vi "Teleop.vi"(10 "Match Info":T5={"Autonomous Elapsed Seconds"=0.0, "TeleOp Elapsed Seconds"=0.0, "Disabled Elapsed Seconds"=0.0, "Visited Autonomous"=FALSE, "Visited TeleOp"=FALSE, "Visited Disabled"=FALSE, "Autonomous Settings"={"Autonomous Style"=enum."Independent", "VI Refnum"=refnum}}, 11 "Call Context":T6) -> ()   [LabVIEW 2020]
doc: "This VI is called for each TeleOp packet received from the DS where the robot is not disabled. It is often used to read from the joysticks and update I/O or to update setpoints for timed control loops. It should complete and return within 20 milliseconds or it may miss DS packets."
uses:
  <vilib>/Rock Robotics/WPI/DriverStation/WPI_DriverStationDerivedRobotMode.ctl
  <vilib>/Rock Robotics/WPI/DriverStation/WPI_DriverStationMatch Info.ctl
  <vilib>/Rock Robotics/WPI/Solenoid/WPI_SolenoidValue.ctl
  <vilib>/Rock Robotics/WPI/ThirdParty/Phoenix-LabVIEW/CANCoder/Controls/CTRE_Phoenix_CANcoder_Faults.ctl
  <vilib>/Rock Robotics/WPI/ThirdParty/Phoenix-LabVIEW/CANCoder/Controls/CTRE_Phoenix_CANcoder_StatusFrame.ctl
  <vilib>/Rock Robotics/WPI/ThirdParty/Phoenix-LabVIEW/Motor Controller/Controls/CTRE_Phoenix_MotorControl_ControlMode.ctl
  <vilib>/Rock Robotics/Network Tables/NT Read Boolean.vi
  <vilib>/Rock Robotics/Network Tables/NT Read Number.vi
  <vilib>/Rock Robotics/WPI/Utilities/WPI_GetSetVariantRefNum.vi
  <vilib>/Rock Robotics/Network Tables/NT Write Boolean Array.vi
  <vilib>/Rock Robotics/Network Tables/NT Write Numeric Array.vi
  <vilib>/Rock Robotics/WPI/Solenoid/WPI_SolenoidSetEnum.vi
  <vilib>/Rock Robotics/WPI/ThirdParty/Phoenix-LabVIEW/CANCoder/Get/CTRE_Phoenix_CANcoder_GetSensorData.vi
  <vilib>/Rock Robotics/WPI/ThirdParty/Phoenix-LabVIEW/Motor Controller/Get/CTRE_Phoenix_MotorController_GetSelectedSensorData.vi
  <vilib>/Rock Robotics/WPI/RobotDrive/WPI_RobotDriveArcadeDrive_Standard(NoSaturation).vi
  <vilib>/Rock Robotics/WPI/ThirdParty/Phoenix-LabVIEW/CANCoder/Set/CTRE_Phoenix_CANcoder_SetPosition.vi
panel:
  out "Talon FX Left Encoder":i32
  out "Talon FX Right Encoder":i32
  out "Right Encoder Position":dbl=-0.5 format="%#_13g"
  out "Left Encoder Position":dbl format="%#_13g"
  out "periodMs":u32=1
  in  "Get status":bool=TRUE
  in  "CANcoder Status Frame":T1=267264 items=["SensorData"=267264, "VbatAndFaults"=267328]
  in  "Period (ms)":u8
  out "In Starting Lvl Seq":bool
  out "In High Lvl Seq":bool
  out "In Ground Lvl Seq":bool
  out "In Mid Lvl Seq":bool
  out "Set Arm Angle Rate":dbl format="%#_13g"
  out "Arm Elevation Position":dbl
  out "Arm Telescope Position":dbl format="%#_13g"
  out "Set Arm Tellescope Rate":dbl
  in  "Arm Tellescope Ground Set Point":dbl=780.0
  in  "Arm Tellescope Allowed Error":dbl=30.0 format="%#_13g"
  in  "Arm Elevation Ground Set Point":dbl=46.0 format="%#_13g"
  in  "Arm Elevation Allowed Error":dbl=3.0 format="%#_13g"
  in  "Arm Tellescope Mid Set Point":dbl=1130.0
  in  "Arm Elevation Mid Setpoint":dbl=80.0 format="%#_13g"
  in  "Arm Tellescope High Set Point":dbl=1790.0
  in  "Arm Elevation High Set Point":dbl=95.0 format="%#_13g"
  in  "Arm Elevation Starting position Set Point":dbl=5.0
  in  "Arm Telescope Starting Set Point":dbl=30.0
  out "Arrived in Set Location":bool
  out "Sticky Faults":T2={"Hardware Fault"=FALSE, "API Error"=FALSE, "Under Voltage"=FALSE, "Reset During Enable"=FALSE, "Magnet Too Weak"=TRUE}
  out "Faults":T3
  in  "Intake value":dbl format="%#_13g"
  in  "Turn Shifter Off":T4=enum."Reverse"
  in  "Shifter Turn On":T4=enum."Forward"
  in  "Break Turn Off":T4=enum."Reverse"
  in  "Break Turn On":T4=enum."Forward"
  out "Sample Slider 0":dbl(slide) scale=0.0..5.0
  out "Sample Boolean 1":bool
  out "Sample Boolean 0":bool
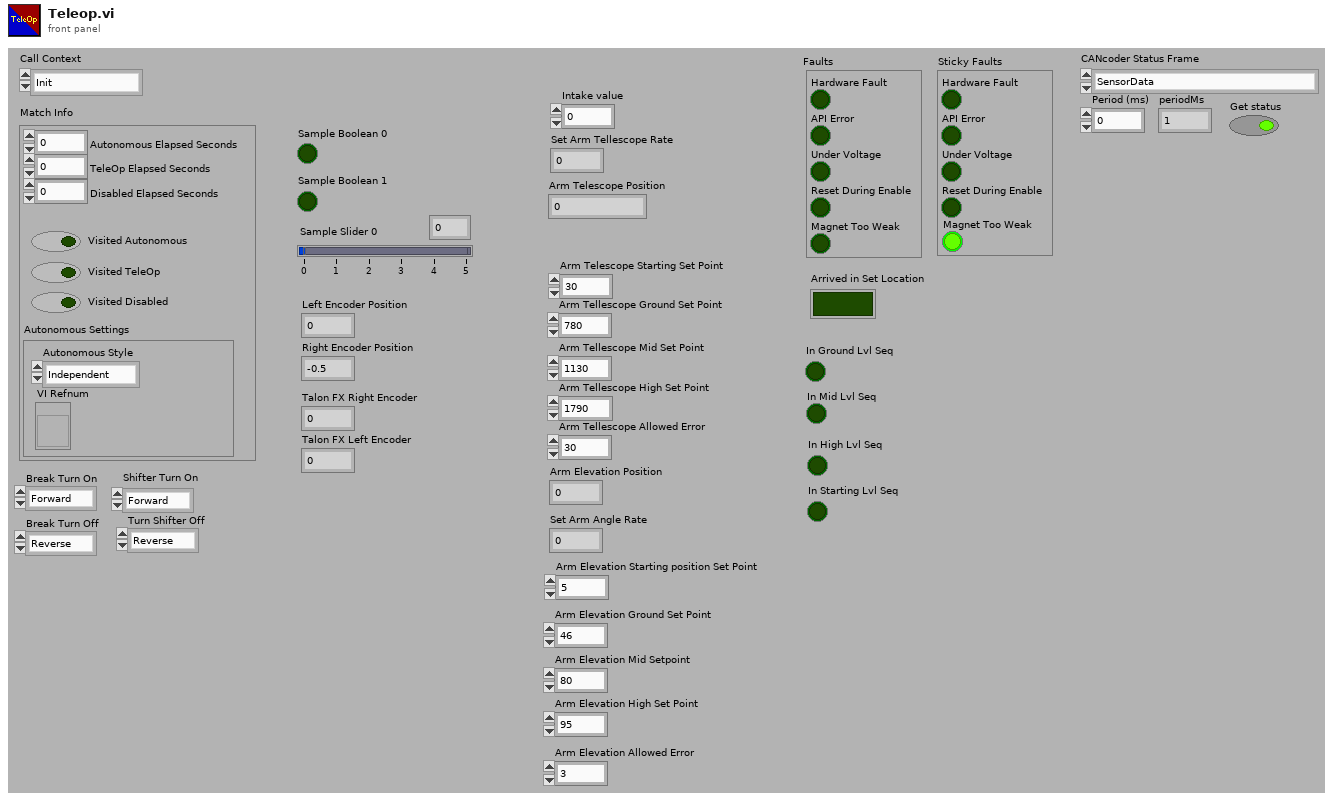
[diagram p1: front panel]
types:
  T1 = typedef "CTRE_Phoenix_CANcoder_StatusFrame.ctl" = u32
  T2 = cluster{"Hardware Fault":bool, "API Error":bool, "Under Voltage":bool, "Reset During Enable":bool, "Magnet Too Weak":bool}
  T3 = typedef "CTRE_Phoenix_CANcoder_Faults.ctl" = cluster{"Hardware Fault":bool, "API Error":bool, "Under Voltage":bool, "Reset During Enable":bool, "Magnet Too Weak":bool}
  T4 = typedef "WPI_SolenoidValue.ctl" = enum16{"Off", "On", "Forward", "Reverse"}
  T5 = typedef "WPI_DriverStationMatch Info.ctl" = cluster{"Autonomous Elapsed Seconds":dbl, "TeleOp Elapsed Seconds":dbl, "Disabled Elapsed Seconds":dbl, "Visited Autonomous":bool, "Visited TeleOp":bool, "Visited Disabled":bool, "Autonomous Settings":cluster{"Autonomous Style":enum16{"Iterative", "Independent"}, "VI Refnum":refnum<vi>}}
  T6 = typedef "WPI_DriverStationDerivedRobotMode.ctl" = enum16{"Init", "Execute", "Stop"}
  T7 = typedef "CTRE_Phoenix_MotorControl_ControlMode.ctl" = u16
  T8 = typedef "CTRE_Phoenix_CANcoder_DeviceRef.ctl" = cluster{"DeviceStatus":errorcluster, "Device Number":u8, "Handle":u64, "UsageFrame":u32, "Library Path":path}
  T9 = typedef "WPI_EncoderDevRef.ctl" = cluster{"DevStatus":errorcluster, "EncoderIndex":T10, "CounterIndex":T11, "DistancePerCount":dbl, "Decoding Type":T12}
  T10 = typedef "FPGA_EncoderIdx.ctl" = enum8{"Enc 0", "Enc 1", "Enc 2", "Enc 3", "Enc 4", "Enc 5", "Enc 6", "Enc 7", "Invalid"}
  T11 = typedef "FPGA_CounterCtrSystemIndex.ctl" = enum8{"Ctr 0", "Ctr 1", "Ctr 2", "Ctr 3", "Ctr 4", "Ctr 5", "Ctr 6", "Ctr 7", "Invalid"}
  T12 = typedef "WPI_EncoderType.ctl" = enum16{"1x", "2x", "4x"}
  T13 = typedef "WPI_MotorControlDeviceRef.ctl" = cluster{"DeviceStatus":errorcluster, "Type":T14, "PWM":cluster{"PWM Channel":T15, "DeadBand":T16}, "CAN":cluster{"Device Number":u8, "SetOutput VI Ref":variant, "GetOutput VI Ref":variant, "Enable VI Ref":variant, "Disable VI Ref":variant, "Data":variant}, "Invert":bool, "DIO PWM":cluster{"PWM \"Enable\" Channel":T15, "DIOChannel":T17, "PWM Rate":dbl}}
  T14 = typedef "WPI_MotorControlType.ctl" = enum16{"PWM", "CAN", "DIO PWM"}
  T15 = typedef "FPGA_DIOPWMChannel.ctl" = enum8{"PWM 0", "PWM 1", "PWM 2", "PWM 3", "PWM 4", "PWM 5", "PWM 6", "PWM 7", "PWM 8", "PWM 9", "PWM MXP 0", "PWM MXP 1", "PWM MXP 2", "PWM MXP 3", "PWM MXP 4", "PWM MXP 5", "PWM MXP 6", "PWM MXP 7", "PWM MXP 8", "PWM MXP 9", "Invalid"}
  T16 = typedef "WPI_PWMDeadband.ctl" = cluster{"Name":string, "maxPositivePwm":i32, "minPositivePwm":i32, "centerPwm":i32, "maxNegativePwm":i32, "minNegativePwm":i32, "angularRange":u16}
  T17 = typedef "FPGA_DIOChannel.ctl" = enum8{"DIO 0", "DIO 1", "DIO 2", "DIO 3", "DIO 4", "DIO 5", "DIO 6", "DIO 7", "DIO 8", "DIO 9", "DIO MXP 0", "DIO MXP 1", "DIO MXP 2", "DIO MXP 3", "DIO MXP 4", "DIO MXP 5", "DIO MXP 6", "DIO MXP 7", "DIO MXP 8", "DIO MXP 9", "DIO MXP 10", "DIO MXP 11", "DIO MXP 12", "DIO MXP 13", "DIO MXP 14", "DIO MXP 15", "SPI Port CS1", "SPI Port CS2", "SPI Port CS3", "SPI Port MISO", "SPI Port MOSI", "Invalid"}
  T18 = typedef "WPI_JoystickDevRef.ctl" = cluster{"Device":T19}
  T19 = typedef "WPI_JoystickDeviceEnum.ctl" = enum16{"USB 0", "USB 1", "USB 2", "USB 3", "USB 4", "USB 5"}
  T20 = typedef "WPI_RobotDriveDevRef.ctl" = cluster{"DevStatus":errorcluster, "Motors[]":T13[], "Square Inputs":bool, "Max Output":dbl}
  T21 = typedef "WPI_ServoDeviceRef.ctl" = cluster{"DeviceStatus":errorcluster, "PWM Channel":T15, "DeadBand":T16}
  T22 = typedef "WPI_SolenoidDevRef.ctl" = cluster{"DevStatus":errorcluster, "Pneumatics Control Module":u8, "Forward Solenoid Channel":T23, "Reverse Solenoid Channel":T23}
  T23 = typedef "WPI_SolenoidChannel.ctl" = enum8{"Solenoid 0", "Solenoid 1", "Solenoid 2", "Solenoid 3", "Solenoid 4", "Solenoid 5", "Solenoid 6", "Solenoid 7", "Solenoid 8", "Solenoid 9", "Solenoid 10", "Solenoid 11", "Solenoid 12", "Solenoid 13", "Solenoid 14", "Solenoid 15", "Invalid"}
  T24 = typedef "WPI_SwitchDevRef.ctl" = cluster{"DevStatus":errorcluster, "DIO Channel":T17, "CntIndex":T11, "Normally Closed":bool}
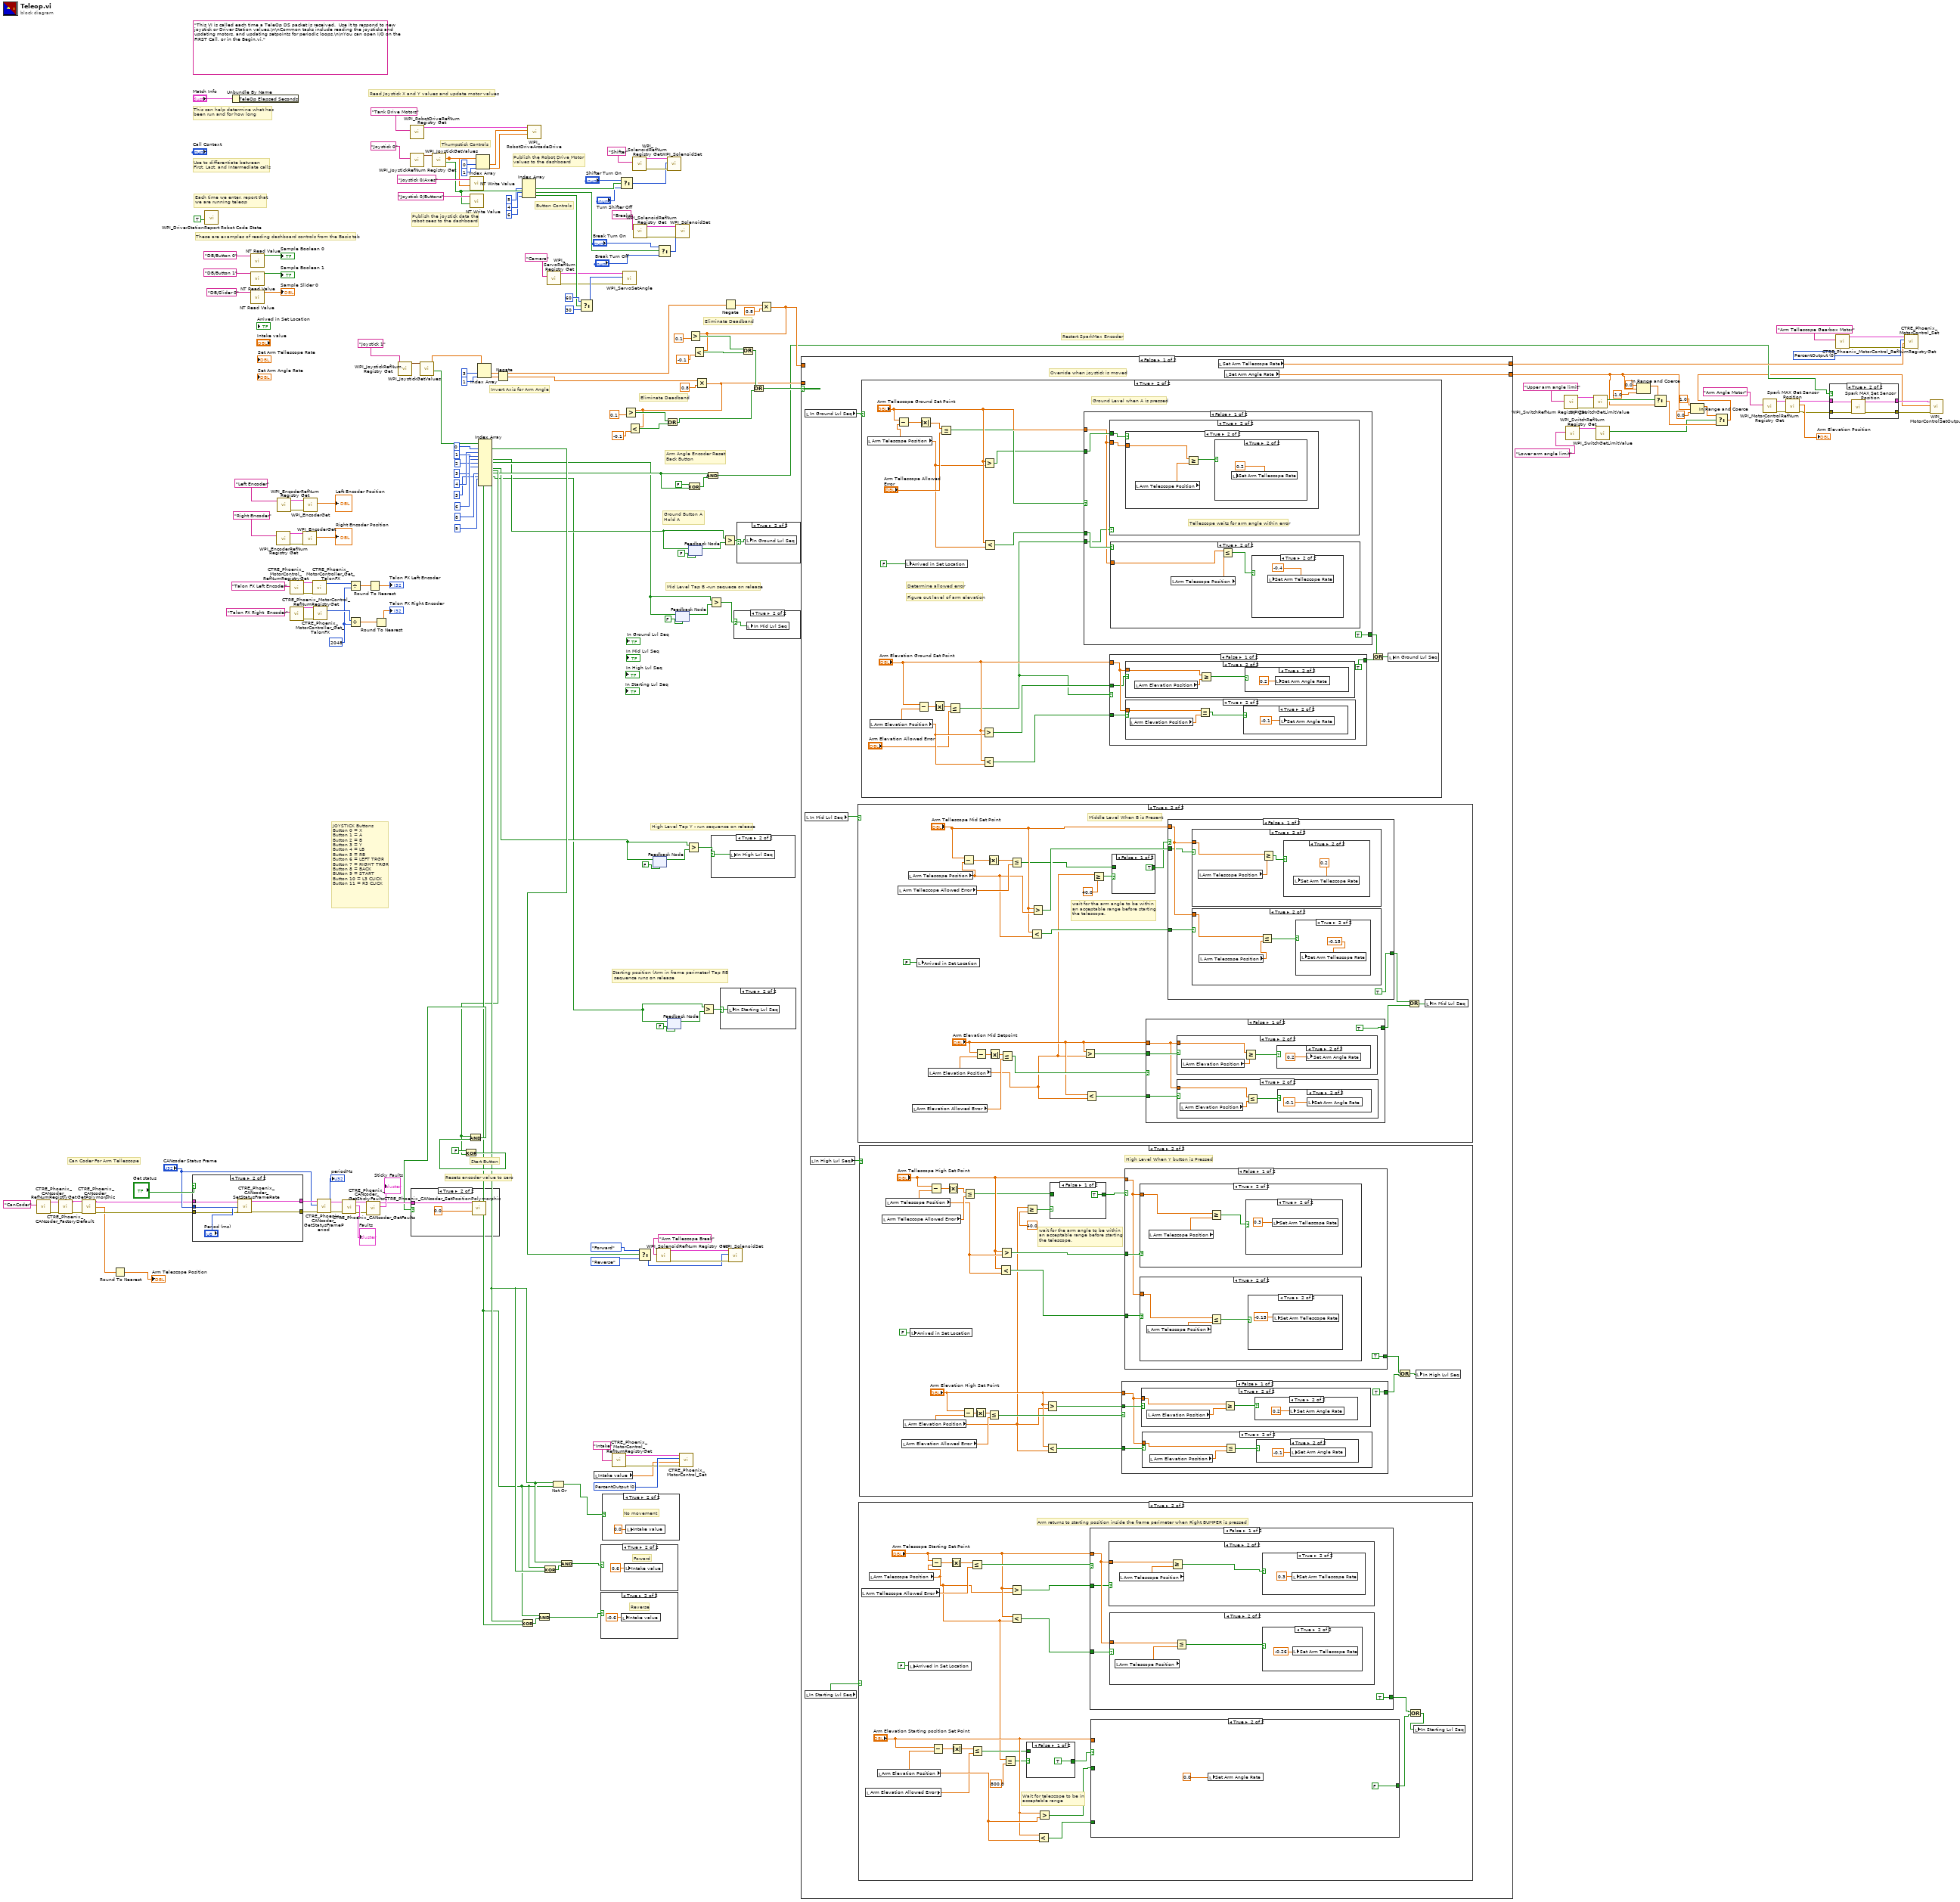
[diagram p0: block diagram]
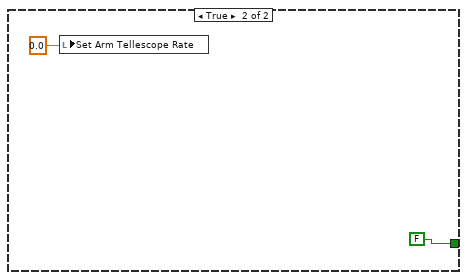
[diagram p15: hidden frame]
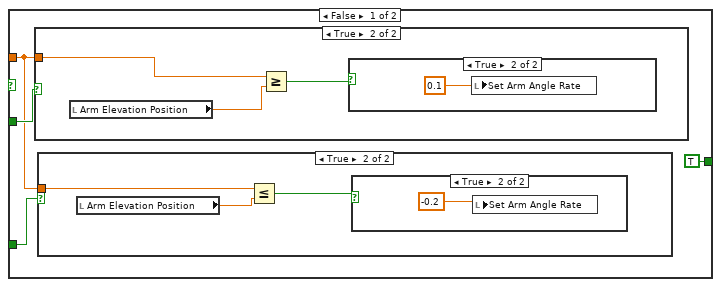
[diagram p16: hidden frame]
diagram:
  w11 = 2048 ("y")
  w144 = T7 0 items=["PercentOutput"=0, "Position"=1, "Velocity"=2, "Current"=3, "Follower"=5, "MotionProfile"=6, "MotionMagic"=7, "MotionProfileArc"=10, "Disabled"=15] ("Control Mode")
  w149 = T7 0 items=["PercentOutput"=0, "Position"=1, "Velocity"=2, "Current"=3, "Follower"=5, "MotionProfile"=6, "MotionMagic"=7, "MotionProfileArc"=10, "Disabled"=15] ("Control Mode")
  (unwired) "This VI is called each time a TeleOp DS packet is received.  Use it to respond to new joystick or Driver Station values.\n\nCommon tasks include reading the joysticks and updating motors, and updating setpoints for periodic loops.\n\nYou can open I/O on the FIRST Call, or in the Begin.vi."
  # "Can Coder For Arm Tellescope"
  # "Starting position (Arm in frame perimeter) Tap RB\n sequence runs on release"
  # "Mid Level Tap B -run sequece on release"
  # "Arm Angle Encoder Reset\nBack Button"
  # "Restart SparkMax Encoder"
  # "Invert Axis for Arm Angle"
  # "Eliminate Deadband"
  # "High Level Tap Y - run sequence on release"
  # "Ground Button A\nHold A"
  # "Start Button"
  # "Resets encoder value to zero"
  # "Eliminate Deadband"
  # "JOYSTICK Buttons\nButton 0 = X\nButton 1 = A\nButton 2 = B\nButton 3 = Y\nButton 4 = LB \nButton 5 = RB\nButton 6 = LEFT TRGR \nButton 7 = RIGHT TRGR \nButton 8 = BACK\nBUtton 9 = START\nButton 10 = L3 CLICK\nButton 11 = R3 CLICK"
  # "Thumpstick Controls"
  # "Button Controls"
  # "Publish the Robot Drive Motor\nvalues to the dashboard"
  # "Publish the joystick data the\nrobot sees to the dashboard"
  # "Read Joystick X and Y values and update motor values"
  # "These are examples of reading dashboard controls from the Basic tab"
  # "Each time we enter, report that\nwe are running teleop"
  # "Use to differentiate between\nFirst, Last, and Intermediate calls"
  # "This can help determine what has\nbeen run and for how long"
  n1 = call <vilib>:"CTRE_Phoenix_CANcoder_RefNumRegistryGet.vi"("refnum name"="CanCoder") -> ("error out"=w41:errorcluster, "CTRE_CANcoder_DeviceRef"=w40:T8)  [unwired: 9 in]
  n2 = call <vilib>:"CTRE_Phoenix_CANcoder_FactoryDefault.vi"("error in"=w41, "CTRE_CANcoder_DeviceRef"=w40) -> ("error out"=w39:errorcluster, "CTRE_CANcoder_DeviceRef"=w38:T8)  [unwired: 8 in]
  n3 = call-poly <vilib>:"CTRE_Phoenix_CANcoder_GetPolymorphic.vi"("CTRE_CANcoder_DeviceRef"=w38, "error in"=w39) -> ("CTRE_CANcoder_DeviceRef"=w36:T8, "Position"=w35:dbl, "error out"=w37:errorcluster)  [unwired: 9 in, 2 out]
  n4 = Round To Nearest(number=w35) -> (nearest integer value=→"Arm Telescope Position":dbl)
  n5 = case shown="True" "Get status" {
    tunnel: w36 -> [w194 w200]
    tunnel: "CANcoder Status Frame" -> [_ w199]
    tunnel: [w194 w197] -> w45
    tunnel: [w193 w196] -> w44
    tunnel: w37 -> [w193 w195]
    frame False {
    }
    frame True {
      n6 = call <vilib>:"CTRE_Phoenix_CANcoder_SetStatusFrameRate.vi"("error in (no error)"=w195, "Period (ms)"="Period (ms)", "CANcoder Status Frame"=w199, "CTRE_CANcoder_DeviceRef"=w200) -> ("error out"=w196:errorcluster, "CTRE_CANcoder_DeviceRef"=w197:T8)  [unwired: 6 in]
    }
  }
  n7 = call <vilib>:"WPI_DriverStationReport Robot Code State.vi"("TeleOp"=TRUE ("Autonomous")) -> ()  [unwired: 10 in, 1 out]
  n8 = Unbundle By Name("Match Info") -> ()  [unwired: 1 out]
  n9 = call-poly <vilib>:"NT Read Value.vi"("name"="DB/Button 0" ("refnum name")) -> ("value"=→"Sample Boolean 0":bool)  [unwired: 8 in, 2 out]
  n10 = call-poly <vilib>:"NT Read Value.vi"("name"="DB/Slider 0" ("refnum name")) -> ("value"=→"Sample Slider 0":dbl)  [unwired: 8 in, 2 out]
  n11 = call-poly <vilib>:"NT Read Value.vi"("name"="DB/Button 1" ("refnum name")) -> ("value"=→"Sample Boolean 1":bool)  [unwired: 8 in, 2 out]
  n12 = call <vilib>:"WPI_EncoderRefNum Registry Get.vi"("refnum name"="Right Encoder") -> ("error out"=w27:errorcluster, "EncoderDevRef"=w26:T9)  [unwired: 9 in]
  n13 = call <vilib>:"WPI_EncoderRefNum Registry Get.vi"("refnum name"="Left Encoder") -> ("error out"=w30:errorcluster, "EncoderDevRef"=w29:T9)  [unwired: 9 in]
  n14 = call <vilib>:"CTRE_Phoenix_MotorControl_RefNumRegistryGet.vi"("refnum name"="Talon FX Left Encoder") -> ("error out"=w18:errorcluster, "PhoenixMotorControlDevRef"=w19:T13)  [unwired: 9 in]
  n15 = call <vilib>:"CTRE_Phoenix_MotorControl_RefNumRegistryGet.vi"("refnum name"="Talon FX Right  Encoder") -> ("error out"=w16:errorcluster, "PhoenixMotorControlDevRef"=w17:T13)  [unwired: 9 in]
  n16 = call <vilib>:"WPI_EncoderGet.vi"("error in (no error)"=w27, "EncoderDevRef"=w26) -> ("Distance"=→"Right Encoder Position":dbl)  [unwired: 4 in, 5 out]
  n17 = call <vilib>:"WPI_EncoderGet.vi"("error in (no error)"=w30, "EncoderDevRef"=w29) -> ("Distance"=→"Left Encoder Position":dbl)  [unwired: 4 in, 5 out]
  n18 = call-poly <vilib>:"CTRE_Phoenix_MotorController_Get_TalonFX.vi"("PhoenixMotorControlDevRef"=w19, "error in"=w18) -> ("Position (Raw Sensor Units)"=w12:i32)  [unwired: 10 in, 3 out]
  n19 = call-poly <vilib>:"CTRE_Phoenix_MotorController_Get_TalonFX.vi"("PhoenixMotorControlDevRef"=w17, "error in"=w16) -> ("Position (Raw Sensor Units)"=w15:i32)  [unwired: 10 in, 3 out]
  n20 = call <vilib>:"CTRE_Phoenix_CANcoder_GetStatusFramePeriod.vi"("error in"=w44, "CANcoder Status Frame"="CANcoder Status Frame", "CTRE_CANcoder_DeviceRef"=w45) -> ("error out"=w31:errorcluster, "periodMs"=→"periodMs":u32, "CTRE_CANcoder_DeviceRef"=w32:T8)  [unwired: 6 in]
  n21 = call <vilib>:"CTRE_Phoenix_CANcoder_GetFaults.vi"("error in"=w31, "CTRE_CANcoder_DeviceRef"=w32) -> ("error out"=w130:errorcluster, "Faults"=→"Faults":T3, "CTRE_CANcoder_DeviceRef"=w131:T8)  [unwired: 7 in]
  n22 = Divide(x=w12, y=w11) -> (x/y=w9:dbl)
  n23 = Divide(x=w15, y=w11) -> (x/y=w14:dbl)
  n24 = call <vilib>:"CTRE_Phoenix_CANcoder_GetStickyFaults.vi"("error in"=w130, "CTRE_CANcoder_DeviceRef"=w131) -> ("Sticky Faults"=→"Sticky Faults":T2, "CTRE_CANcoder_DeviceRef"=w114:T8)  [unwired: 7 in, 1 out]
  n25 = Round To Nearest(number=w9) -> (nearest integer value=→"Talon FX Left Encoder":dbl)
  n26 = Round To Nearest(number=w14) -> (nearest integer value=→"Talon FX Right Encoder":dbl)
  n27 = call <vilib>:"WPI_JoystickRefNum Registry Get.vi"("refnum name"="Joystick 1") -> ("JoystickDevRef"=w154:T18)  [unwired: 1 in, 9 out]
  n28 = call <vilib>:"WPI_RobotDriveRefNum Registry Get.vi"("refnum name"="Tank Drive Motors") -> ("RobotDriveDevRef"=w177:T20)  [unwired: 1 in, 9 out]
  n29 = call <vilib>:"WPI_JoystickRefNum Registry Get.vi"("refnum name"="Joystick 0") -> ("JoystickDevRef"=w183:T18)  [unwired: 1 in, 9 out]
  n30 = call <vilib>:"WPI_JoystickGetValues.vi"("JoystickDevRef"=w154) -> ("Buttons"=w150:bool[], "Axes"=w146:dbl[])  [unwired: 6 in, 3 out]
  n31 = call <vilib>:"WPI_JoystickGetValues.vi"("JoystickDevRef"=w183) -> ("Buttons"=w167:bool[], "Axes"=w180:dbl[])  [unwired: 6 in, 3 out]
  n32 = call-poly <vilib>:"NT Write Value.vi"("value"=w180, "name"="Joystick 0/Axes" ("Name")) -> ()  [unwired: 9 in, 1 out]
  n33 = call-poly <vilib>:"NT Write Value.vi"("value"=w167, "name"="Joystick 0/Buttons" ("Name")) -> ()  [unwired: 9 in, 1 out]
  n34 = Index Array(array=w180, index #1=0 ("index"), index #2=1 ("index")) -> (element #1=w176:dbl, element #2=w175:dbl)
  n35 = Index Array "Index Array"(array=w146, index #1=3 ("index"), index #2=1 ("index")) -> (element #1=w118:dbl, element #2=w97:dbl)
  n36 = Index Array "Index Array"(array=w150, index #1=0 ("index"), index #2=4 ("index"), index #3=6 ("index"), index #4=1 ("index"), index #5=2 ("index"), index #6=3 ("index"), index #7=9 ("index"), index #8=8 ("index"), index #9=5) -> (element #1=w115:bool, element #2=w108:bool, element #3=w107:bool, element #4=w73:bool, element #5=w77:bool, element #6=w69:bool, element #7=w103:bool, element #8=w83:bool, element #9=w65:bool)  [unwired: 2 in, 2 out]
  n37 = Exclusive Or(1:w103, 2:FALSE ("x")) -> (0:w116:bool)
  n38 = And(x=w103, y=w116) -> (x .and. y?=w113:bool)
  n39 = case shown="True" w113 {
    tunnel: w114 -> [_ w202]
    frame False {
    }
    frame True {
      n40 = call-poly <vilib>:"CTRE_Phoenix_CANcoder_SetPositionPolymorphic.vi"("Position"=0.0, "CTRE_CANcoder_DeviceRef"=w202) -> ()  [unwired: 8 in, 2 out]
    }
  }
  n41 = Negate(x=w97) -> (-x=w47:dbl)
  n42 = Exclusive Or(1:w107, 2:w108) -> (0:w137:bool)
  n43 = Index Array(array=w167, index #1=5 ("index"), index #2=4 ("index"), index #3=6 ("index")) -> (element #1=w162:bool, element #2=w166:bool, element #3=w4:bool)
  n44 = call-poly <vilib>:"WPI_RobotDriveArcadeDrive.vi"("Y axis value"=w175, "X axis value"=w176, "RobotDriveDevRef"=w177) -> ()  [unwired: 6 in, 3 out]
  n45 = And(x=w107, y=w137) -> (x .and. y?=w136:bool)
  n46 = Exclusive Or(1:w108, 2:w107) -> (0:w135:bool)
  n47 = call <vilib>:"WPI_ServoRefNum Registry Get.vi"("refnum name"="Camara") -> ("error out"=w3:errorcluster, "ServoDeviceRef"=w2:T21)  [unwired: 9 in]
  n48 = Not Or(1:w107, 2:w108) -> (0:w133:bool)
  n49 = And(x=w108, y=w135) -> (x .and. y?=w134:bool)
  n50 = Select(t=60, s=w4, f=30) -> (s? t:f=w7:i32)
  n51 = local read "Intake value"() -> (w140:dbl)
  n52 = case shown="True" w136 {
    frame False {
    }
    frame True {
      # "Reverse"
      n53 = local write "Intake value"(-0.6 ("Intake value")) -> ()
    }
  }
  n54 = case shown="True" w134 {
    frame False {
    }
    frame True {
      # "Foward"
      n55 = local write "Intake value"(0.6 ("Intake value")) -> ()
    }
  }
  n56 = case shown="True" w133 {
    frame False {
    }
    frame True {
      # "No movement"
      n57 = local write "Intake value"(0.0 ("Intake value")) -> ()
    }
  }
  n58 = call <vilib>:"CTRE_Phoenix_MotorControl_RefNumRegistryGet.vi"("refnum name"="Intake") -> ("error out"=w142:errorcluster, "PhoenixMotorControlDevRef"=w143:T13)  [unwired: 9 in]
  n59 = Select(t="Shifter Turn On", s=w162, f="Turn Shifter Off") -> (s? t:f=w157:T4)
  n60 = call <vilib>:"WPI_ServoSetAngle.vi"("error in (no error)"=w3, "Angle"=w7, "ServoDeviceRef"=w2) -> ()  [unwired: 7 in, 2 out]
  n61 = call <vilib>:"WPI_SolenoidRefNum Registry Get.vi"("refnum name"="Shifter") -> ("error out"=w173:errorcluster, "SolenoidDevRef"=w174:T22)  [unwired: 9 in]
  n62 = call <vilib>:"WPI_SolenoidRefNum Registry Get.vi"("refnum name"="Breaks") -> ("error out"=w169:errorcluster, "SolenoidDevRef"=w168:T22)  [unwired: 9 in]
  n63 = Select(t=WPI_SolenoidValue."Forward" ("Value"), s=w115, f=WPI_SolenoidValue."Reverse" ("Value")) -> (s? t:f=w125:T4)
  n64 = feedback #1(FALSE) -> (w71:bool)
  n65 = feedback-in #1(w69) -> ()
  n66 = call <vilib>:"WPI_SolenoidRefNum Registry Get.vi"("refnum name"="Arm Tellescope Break") -> ("error out"=w152:errorcluster, "SolenoidDevRef"=w156:T22)  [unwired: 9 in]
  n67 = Select(t="Break Turn On", s=w166, f="Break Turn Off") -> (s? t:f=w170:T4)
  n68 = call-poly <vilib>:"WPI_SolenoidSet.vi"("error in (no error)"=w173, "Value"=w157, "SolenoidDevRef"=w174) -> ()  [unwired: 7 in, 2 out]
  n69 = feedback #2(FALSE) -> (w67:bool)
  n70 = feedback-in #2(w65) -> ()
  n71 = feedback #3(FALSE) -> (w79:bool)
  n72 = feedback-in #3(w77) -> ()
  n73 = call-poly <vilib>:"WPI_SolenoidSet.vi"("error in (no error)"=w169, "Value"=w170, "SolenoidDevRef"=w168) -> ()  [unwired: 7 in, 2 out]
  n74 = call <vilib>:"CTRE_Phoenix_MotorControl_Set.vi"("error in (no error)"=w142, "Output"=w140, "Control Mode"=w144, "PhoenixMotorControlDevRef"=w143) -> ()  [unwired: 6 in, 2 out]
  n75 = Greater?(x=w69, y=w71) -> (0:w68:bool)
  n76 = Exclusive Or(1:w83, 2:FALSE ("x")) -> (0:w84:bool)
  n77 = feedback #4(FALSE) -> (w75:bool)
  n78 = feedback-in #4(w73) -> ()
  n79 = Multiply(x=w47, y=0.8) -> (x*y=w93:dbl)
  n80 = Greater?(x=w93, y=0.1) -> (0:w99:bool)
  n81 = Less?(x=w93, y=-0.1) -> (x < y?=w100:bool)
  n82 = Or(x=w99, y=w100) -> (x .or. y?=w96:bool)
  n83 = Greater?(x=w65, y=w67) -> (0:w64:bool)
  n84 = And(x=w83, y=w84) -> (x .and. y?=w81:bool)
  n85 = Greater?(x=w77, y=w79) -> (0:w76:bool)
  n86 = case shown="True" w68 {
    selector: w68 -> [_ w206]
    frame False {
    }
    frame True {
      n87 = local write "In High Lvl Seq"(w206) -> ()
    }
  }
  n88 = case shown="True" w64 {
    selector: w64 -> [_ w207]
    frame False {
    }
    frame True {
      n89 = local write "In Starting Lvl Seq"(w207) -> ()
    }
  }
  n90 = Greater?(x=w73, y=w75) -> (0:w72:bool)
  n91 = Negate(x=w118) -> (-x=w124:dbl)
  n92 = call-poly <vilib>:"WPI_SolenoidSet.vi"("error in (no error)"=w152, "Value"=w125, "SolenoidDevRef"=w156) -> ()  [unwired: 7 in, 2 out]
  n93 = case shown="True" w76 {
    selector: w76 -> [_ w208]
    frame False {
    }
    frame True {
      n94 = local write "In Mid Lvl Seq"(w208) -> ()
    }
  }
  n95 = case shown="True" w72 {
    selector: w72 -> [_ w209]
    frame False {
    }
    frame True {
      n96 = local write "In Ground Lvl Seq"(w209) -> ()
    }
  }
  n97 = Multiply(x=w124, y=0.8) -> (x*y=w105:dbl)
  n98 = Greater?(x=w105, y=0.1) -> (0:w120:bool)
  n99 = Less?(x=w105, y=-0.1) -> (x < y?=w121:bool)
  n100 = Or(x=w120, y=w121) -> (x .or. y?=w95:bool)
  n101 = Or(x=w95, y=w96) -> (x .or. y?=w94:bool)
  n102 = case shown="False" w94 {
    tunnel: w105 -> [_ w428]
    tunnel: [w215 w428] -> w104
    tunnel: w93 -> [_ w427]
    tunnel: [w214 w427] -> w51
    frame False {
      # "Override when joystick is moved"
      n103 = local read "In Starting Lvl Seq"() -> (w210:bool)
      n104 = local read "In Ground Lvl Seq"() -> (w212:bool)
      n105 = local read "In Mid Lvl Seq"() -> (w213:bool)
      n106 = local read "In High Lvl Seq"() -> (w211:bool)
      n107 = case shown="True" w213 {
        frame False {
        }
        frame True {
          # "wait for the arm angle to be within\nan acceptable range before starting \nthe telescope."
          # "Middle Level When B is Present"
          n108 = local read "Arm Tellescope Allowed Error"() -> (w342:dbl)
          n109 = local read "Arm Telescope Position"() -> (w338:dbl)
          n110 = local read "Arm Elevation Allowed Error"() -> (w332:dbl)
          n111 = local write "Arrived in Set Location"(FALSE) -> ()
          n112 = local read "Arm Elevation Position"() -> (w322:dbl)
          n113 = Subtract(x="Arm Tellescope Mid Set Point", y=w338) -> (x-y=w344:dbl)
          n114 = Subtract(x="Arm Elevation Mid Setpoint", y=w322) -> (x-y=w337:dbl)
          n115 = Absolute Value(x=w344) -> (abs(x)=w343:dbl)
          n116 = Absolute Value(x=w337) -> (abs(x)=w336:dbl)
          n117 = Less Or Equal?(x=w336, y=w332) -> (x <= y?=w333:bool)
          n118 = Less Or Equal?(x=w343, y=w342) -> (x <= y?=w327:bool)
          n119 = Less?(x="Arm Tellescope Mid Set Point", y=w338) -> (x < y?=w340:bool)
          n120 = Greater?(x="Arm Tellescope Mid Set Point", y=w338) -> (0:w339:bool)
          n121 = Greater?(x="Arm Elevation Mid Setpoint", y=w322) -> (0:w334:bool)
          n122 = Less?(x="Arm Elevation Mid Setpoint", y=w322) -> (x < y?=w335:bool)
          n123 = Greater Or Equal?(x=w322, y=40.0) -> (x >= y?=w325:bool)
          n124 = case shown="False" w325 {
            tunnel: w327 -> [_ w346]
            tunnel: [TRUE w346] -> w326
            frame False {
            }
            frame True {
            }
          }
          n125 = case shown="False" w333 {
            tunnel: w335 -> [w350 _]
            tunnel: w334 -> [w349 _]
            tunnel: "Arm Elevation Mid Setpoint" -> [w348 _]
            tunnel: [TRUE FALSE] -> w329
            frame False {
              n126 = case shown="True" w349 {
                tunnel: w348 -> [_ w355]
                frame False {
                }
                frame True {
                  n127 = local read "Arm Elevation Position"() -> (w356:dbl)
                  n128 = Greater Or Equal?(x=w355, y=w356) -> (x >= y?=w357:bool)
                  n129 = case shown="True" w357 {
                    frame False {
                    }
                    frame True {
                      n130 = local write "Set Arm Angle Rate"(0.2) -> ()
                    }
                  }
                }
              }
              n131 = case shown="True" w350 {
                tunnel: w348 -> [_ w351]
                frame False {
                }
                frame True {
                  n132 = local read "Arm Elevation Position"() -> (w352:dbl)
                  n133 = Less Or Equal?(x=w351, y=w352) -> (x <= y?=w353:bool)
                  n134 = case shown="True" w353 {
                    frame False {
                    }
                    frame True {
                      n135 = local write "Set Arm Angle Rate"(-0.1) -> ()
                    }
                  }
                }
              }
            }
            frame True {
              n136 = local write "Set Arm Angle Rate"(0.0) -> ()
            }
          }
          n137 = case shown="False" w326 {
            tunnel: "Arm Tellescope Mid Set Point" -> [w364 _]
            tunnel: w340 -> [w363 _]
            tunnel: w339 -> [w362 _]
            tunnel: [TRUE ("Start Mid Lvl Seq") FALSE ("Start Mid Lvl Seq")] -> w330
            frame False {
              n138 = case shown="True" w362 {
                tunnel: w364 -> [_ w370]
                frame False {
                }
                frame True {
                  n139 = local read "Arm Telescope Position"() -> (w371:dbl)
                  n140 = Greater Or Equal?(x=w370, y=w371) -> (x >= y?=w369:bool)
                  n141 = case shown="True" w369 {
                    frame False {
                    }
                    frame True {
                      n142 = local write "Set Arm Tellescope Rate"(0.2) -> ()
                    }
                  }
                }
              }
              n143 = case shown="True" w363 {
                tunnel: w364 -> [_ w365]
                frame False {
                }
                frame True {
                  n144 = local read "Arm Telescope Position"() -> (w366:dbl)
                  n145 = Less Or Equal?(x=w365, y=w366) -> (x <= y?=w367:bool)
                  n146 = case shown="True" w367 {
                    frame False {
                    }
                    frame True {
                      n147 = local write "Set Arm Tellescope Rate"(-0.15) -> ()
                    }
                  }
                }
              }
            }
            frame True {
              n148 = local write "Set Arm Tellescope Rate"(0.0) -> ()
            }
          }
          n149 = Or(x=w330, y=w329) -> (x .or. y?=w331:bool)
          n150 = local write "In Mid Lvl Seq"(w331) -> ()
        }
      }
      n151 = case shown="True" w210 {
        frame False {
        }
        frame True {
          # "Wait for telescope to be in \nacceptable range"
          # "Arm returns to starting position inside the frame perimeter when Right BUMPER is pressed"
          n152 = local read "Arm Tellescope Allowed Error"() -> (w230:dbl)
          n153 = local read "Arm Elevation Allowed Error"() -> (w235:dbl)
          n154 = local read "Arm Telescope Position"() -> (w216:dbl)
          n155 = local read "Arm Elevation Position"() -> (w236:dbl)
          n156 = local write "Arrived in Set Location"(FALSE ("Arrived in Set Location")) -> ()
          n157 = Subtract(x="Arm Telescope Starting Set Point", y=w216) -> (x-y=w232:dbl)
          n158 = Subtract(x="Arm Elevation Starting position Set Point", y=w236) -> (x-y=w238:dbl)
          n159 = Absolute Value(x=w232) -> (abs(x)=w231:dbl)
          n160 = Absolute Value(x=w238) -> (abs(x)=w237:dbl)
          n161 = Less Or Equal?(x=w231, y=w230) -> (x <= y?=w229:bool)
          n162 = Less Or Equal?(x=w237, y=w235) -> (x <= y?=w219:bool)
          n163 = Less Or Equal?(x=w216, y=800.0) -> (x <= y?=w218:bool)
          n164 = Greater?(x="Arm Telescope Starting Set Point", y=w216) -> (0:w227:bool)
          n165 = Less?(x="Arm Telescope Starting Set Point", y=w216) -> (x < y?=w226:bool)
          n166 = case shown="False" w218 {
            tunnel: [TRUE w240] -> w220
            tunnel: w219 -> [_ w240]
            frame False {
            }
            frame True {
            }
          }
          n167 = Less?(x="Arm Elevation Starting position Set Point", y=w236) -> (x < y?=w233:bool)
          n168 = Greater?(x="Arm Elevation Starting position Set Point", y=w236) -> (0:w221:bool)
          n169 = case shown="False" w229 {
            tunnel: "Arm Telescope Starting Set Point" -> [w244 _]
            tunnel: w227 -> [w243 _]
            tunnel: w226 -> [w242 _]
            tunnel: [TRUE FALSE] -> w223
            frame False {
              n170 = case shown="True" w243 {
                tunnel: w244 -> [_ w251]
                frame False {
                }
                frame True {
                  n171 = local read "Arm Telescope Position"() -> (w250:dbl)
                  n172 = Greater Or Equal?(x=w251, y=w250) -> (x >= y?=w249:bool)
                  n173 = case shown="True" w249 {
                    frame False {
                    }
                    frame True {
                      n174 = local write "Set Arm Tellescope Rate"(0.3) -> ()
                    }
                  }
                }
              }
              n175 = case shown="True" w242 {
                tunnel: w244 -> [_ w247]
                frame False {
                }
                frame True {
                  n176 = local read "Arm Telescope Position"() -> (w246:dbl)
                  n177 = Less Or Equal?(x=w247, y=w246) -> (x <= y?=w245:bool)
                  n178 = case shown="True" w245 {
                    frame False {
                    }
                    frame True {
                      n179 = local write "Set Arm Tellescope Rate"(-0.26) -> ()
                    }
                  }
                }
              }
            }
            frame True {
              n180 = local write "Set Arm Tellescope Rate"(0.0) -> ()
            }
          }
          n181 = case shown="True" w220 {
            tunnel: "Arm Elevation Starting position Set Point" -> [w256 _]
            tunnel: w233 -> [w258 _]
            tunnel: w221 -> [w257 _]
            tunnel: [TRUE FALSE] -> w222
            frame False {
              n182 = case shown="True" w257 {
                tunnel: w256 -> [_ w264]
                frame False {
                }
                frame True {
                  n183 = local read "Arm Elevation Position"() -> (w265:dbl)
                  n184 = Greater Or Equal?(x=w264, y=w265) -> (x >= y?=w263:bool)
                  n185 = case shown="True" w263 {
                    frame False {
                    }
                    frame True {
                      n186 = local write "Set Arm Angle Rate"(0.1) -> ()
                    }
                  }
                }
              }
              n187 = case shown="True" w258 {
                tunnel: w256 -> [_ w261]
                frame False {
                }
                frame True {
                  n188 = local read "Arm Elevation Position"() -> (w260:dbl)
                  n189 = Less Or Equal?(x=w261, y=w260) -> (x <= y?=w259:bool)
                  n190 = case shown="True" w259 {
                    frame False {
                    }
                    frame True {
                      n191 = local write "Set Arm Angle Rate"(-0.2) -> ()
                    }
                  }
                }
              }
            }
            frame True {
              n192 = local write "Set Arm Angle Rate"(0.0) -> ()
            }
          }
          n193 = Or(x=w223, y=w222) -> (x .or. y?=w224:bool)
          n194 = local write "In Starting Lvl Seq"(w224) -> ()
        }
      }
      n195 = case shown="True" w211 {
        frame False {
        }
        frame True {
          # "wait for the arm angle to be within\nan acceptable range before starting \nthe telescope."
          # "High Level When Y button is Pressed"
          n196 = local read "Arm Tellescope Allowed Error"() -> (w289:dbl)
          n197 = local read "Arm Telescope Position"() -> (w286:dbl)
          n198 = local read "Arm Elevation Allowed Error"() -> (w281:dbl)
          n199 = local read "Arm Elevation Position"() -> (w270:dbl)
          n200 = local write "Arrived in Set Location"(FALSE ("Arrived in Set Location")) -> ()
          n201 = Subtract(x="Arm Tellescope High Set Point", y=w286) -> (x-y=w291:dbl)
          n202 = Absolute Value(x=w291) -> (abs(x)=w290:dbl)
          n203 = Subtract(x="Arm Elevation High Set Point", y=w270) -> (x-y=w284:dbl)
          n204 = Less Or Equal?(x=w290, y=w289) -> (x <= y?=w272:bool)
          n205 = Absolute Value(x=w284) -> (abs(x)=w283:dbl)
          n206 = Less Or Equal?(x=w283, y=w281) -> (x <= y?=w282:bool)
          n207 = Less?(x="Arm Tellescope High Set Point", y=w286) -> (x < y?=w287:bool)
          n208 = Greater?(x="Arm Tellescope High Set Point", y=w286) -> (0:w288:bool)
          n209 = Greater Or Equal?(x=w270, y=40.0) -> (x >= y?=w271:bool)
          n210 = Greater?(x="Arm Elevation High Set Point", y=w270) -> (0:w279:bool)
          n211 = Less?(x="Arm Elevation High Set Point", y=w270) -> (x < y?=w280:bool)
          n212 = case shown="False" w271 {
            tunnel: [TRUE w293] -> w273
            tunnel: w272 -> [_ w293]
            frame False {
            }
            frame True {
            }
          }
          n213 = case shown="False" w282 {
            tunnel: w280 -> [w297 _]
            tunnel: w279 -> [w296 _]
            tunnel: "Arm Elevation High Set Point" -> [w295 _]
            tunnel: [TRUE FALSE] -> w274
            frame False {
              n214 = case shown="True" w296 {
                tunnel: w295 -> [_ w302]
                frame False {
                }
                frame True {
                  n215 = local read "Arm Elevation Position"() -> (w303:dbl)
                  n216 = Greater Or Equal?(x=w302, y=w303) -> (x >= y?=w304:bool)
                  n217 = case shown="True" w304 {
                    frame False {
                    }
                    frame True {
                      n218 = local write "Set Arm Angle Rate"(0.2) -> ()
                    }
                  }
                }
              }
              n219 = case shown="True" w297 {
                tunnel: w295 -> [_ w298]
                frame False {
                }
                frame True {
                  n220 = local read "Arm Elevation Position"() -> (w299:dbl)
                  n221 = Less Or Equal?(x=w298, y=w299) -> (x <= y?=w300:bool)
                  n222 = case shown="True" w300 {
                    frame False {
                    }
                    frame True {
                      n223 = local write "Set Arm Angle Rate"(-0.1) -> ()
                    }
                  }
                }
              }
            }
            frame True {
              n224 = local write "Set Arm Angle Rate"(0.0) -> ()
            }
          }
          n225 = case shown="False" w273 {
            tunnel: w288 -> [w311 _]
            tunnel: w287 -> [w310 _]
            tunnel: "Arm Tellescope High Set Point" -> [w309 _]
            tunnel: [TRUE FALSE] -> w275
            frame False {
              n226 = case shown="True" w311 {
                tunnel: w309 -> [_ w317]
                frame False {
                }
                frame True {
                  n227 = local read "Arm Telescope Position"() -> (w316:dbl)
                  n228 = Greater Or Equal?(x=w317, y=w316) -> (x >= y?=w318:bool)
                  n229 = case shown="True" w318 {
                    frame False {
                    }
                    frame True {
                      n230 = local write "Set Arm Tellescope Rate"(0.3) -> ()
                    }
                  }
                }
              }
              n231 = case shown="True" w310 {
                tunnel: w309 -> [_ w313]
                frame False {
                }
                frame True {
                  n232 = local read "Arm Telescope Position"() -> (w312:dbl)
                  n233 = Less Or Equal?(x=w313, y=w312) -> (x <= y?=w314:bool)
                  n234 = case shown="True" w314 {
                    frame False {
                    }
                    frame True {
                      n235 = local write "Set Arm Tellescope Rate"(-0.15) -> ()
                    }
                  }
                }
              }
            }
            frame True {
              n236 = local write "Set Arm Tellescope Rate"(0.0) -> ()
            }
          }
          n237 = Or(x=w275, y=w274) -> (x .or. y?=w276:bool)
          n238 = local write "In High Lvl Seq"(w276) -> ()
        }
      }
      n239 = case shown="True" w212 {
        frame False {
        }
        frame True {
          # "Determine allowed error"
          # "Figure out level of arm elevation"
          # "Ground Level when A is pressed"
          n240 = local read "Arm Telescope Position"() -> (w389:dbl)
          n241 = local read "Arm Elevation Position"() -> (w383:dbl)
          n242 = Subtract(x="Arm Tellescope Ground Set Point", y=w389) -> (x-y=w392:dbl)
          n243 = local write "Arrived in Set Location"(FALSE) -> ()
          n244 = Subtract(x="Arm Elevation Ground Set Point", y=w383) -> (x-y=w388:dbl)
          n245 = Absolute Value(x=w392) -> (abs(x)=w391:dbl)
          n246 = Absolute Value(x=w388) -> (abs(x)=w387:dbl)
          n247 = Less Or Equal?(x=w391, y="Arm Tellescope Allowed Error") -> (x <= y?=w381:bool)
          n248 = Less Or Equal?(x=w387, y="Arm Elevation Allowed Error") -> (x <= y?=w378:bool)
          n249 = Greater?(x="Arm Elevation Ground Set Point", y=w383) -> (0:w385:bool)
          n250 = Less?(x="Arm Elevation Ground Set Point", y=w383) -> (x < y?=w384:bool)
          n251 = Greater?(x="Arm Tellescope Ground Set Point", y=w389) -> (0:w380:bool)
          n252 = Less?(x="Arm Tellescope Ground Set Point", y=w389) -> (x < y?=w379:bool)
          n253 = case shown="False" w381 {
            tunnel: w380 -> [w399 _]
            tunnel: w379 -> [w398 _]
            tunnel: "Arm Tellescope Ground Set Point" -> [w397 _]
            tunnel: w378 -> [w396 _]
            tunnel: [TRUE FALSE] -> w376
            frame False {
              n254 = case shown="True" w396 {
                tunnel: w399 -> [_ w401]
                tunnel: w397 -> [_ w400]
                frame False {
                }
                frame True {
                  # "Tellescope waits for arm angle within error"
                  n255 = case shown="True" w401 {
                    tunnel: w400 -> [_ w402]
                    frame False {
                    }
                    frame True {
                      n256 = local read "Arm Telescope Position"() -> (w404:dbl)
                      n257 = Greater Or Equal?(x=w402, y=w404) -> (x >= y?=w403:bool)
                      n258 = case shown="True" w403 {
                        frame False {
                        }
                        frame True {
                          n259 = local write "Set Arm Tellescope Rate"(0.2 ("Position Telloscoping arm")) -> ()
                        }
                      }
                    }
                  }
                }
              }
              n260 = case shown="True" w398 {
                tunnel: w397 -> [_ w406]
                frame False {
                }
                frame True {
                  n261 = local read "Arm Telescope Position"() -> (w408:dbl)
                  n262 = Less Or Equal?(x=w406, y=w408) -> (x <= y?=w407:bool)
                  n263 = case shown="True" w407 {
                    frame False {
                    }
                    frame True {
                      n264 = local write "Set Arm Tellescope Rate"(-0.4 ("Arm Movement")) -> ()
                    }
                  }
                }
              }
            }
            frame True {
              n265 = local write "Set Arm Tellescope Rate"(0.0 ("Arm Tellescope Set Value")) -> ()
            }
          }
          n266 = case shown="False" w378 {
            tunnel: "Arm Elevation Ground Set Point" -> [w415 _]
            tunnel: w385 -> [w414 _]
            tunnel: w384 -> [w413 _]
            tunnel: [TRUE FALSE] -> w375
            frame False {
              n267 = case shown="True" w414 {
                tunnel: w415 -> [_ w420]
                frame False {
                }
                frame True {
                  n268 = local read "Arm Elevation Position"() -> (w421:dbl)
                  n269 = Greater Or Equal?(x=w420, y=w421) -> (x >= y?=w422:bool)
                  n270 = case shown="True" w422 {
                    frame False {
                    }
                    frame True {
                      n271 = local write "Set Arm Angle Rate"(0.2) -> ()
                    }
                  }
                }
              }
              n272 = case shown="True" w413 {
                tunnel: w415 -> [_ w416]
                frame False {
                }
                frame True {
                  n273 = local read "Arm Elevation Position"() -> (w417:dbl)
                  n274 = Less Or Equal?(x=w416, y=w417) -> (x <= y?=w418:bool)
                  n275 = case shown="True" w418 {
                    frame False {
                    }
                    frame True {
                      n276 = local write "Set Arm Angle Rate"(-0.1) -> ()
                    }
                  }
                }
              }
            }
            frame True {
              n277 = local write "Set Arm Angle Rate"(0.0 ("Set Arm Elevation Rate")) -> ()
            }
          }
          n278 = Or(x=w376, y=w375) -> (x .or. y?=w377:bool)
          n279 = local write "In Ground Lvl Seq"(w377) -> ()
        }
      }
      n280 = local read "Set Arm Tellescope Rate"() -> (w215:dbl)
      n281 = local read "Set Arm Angle Rate"() -> (w214:dbl)
    }
    frame True {
      # "Give Control To Driver Joystick"
      n282 = local write "In Mid Lvl Seq"(FALSE ("Start Mid Lvl Seq")) -> ()
    }
  }
  n283 = call <vilib>:"WPI_SwitchRefNum Registry Get.vi"("refnum name"="Upper arm angle limit") -> ("error out"=w62:errorcluster, "SwitchDevRef"=w61:T24)  [unwired: 9 in]
  n284 = call <vilib>:"WPI_SwitchRefNum Registry Get.vi"("refnum name"="Lower arm angle limit") -> ("SwitchDevRef"=w63:T24)  [unwired: 9 in, 1 out]
  n285 = call <vilib>:"WPI_SwitchGetLimitValue.vi"("error in (no error)"=w62, "SwitchDevRef"=w61) -> ("Switch Pressed"=w60:bool)  [unwired: 7 in, 2 out]
  n286 = call <vilib>:"WPI_SwitchGetLimitValue.vi"("SwitchDevRef"=w63) -> ("Switch Pressed"=w52:bool)  [unwired: 8 in, 2 out]
  n287 = In Range and Coerce(upper limit=0.0, x=w51, lower limit=-1.0) -> (coerced(x)=w59:dbl)  [unwired: 1 out]
  n288 = Select(t=w59, s=w60, f=w51) -> (s? t:f=w54:dbl)
  n289 = In Range and Coerce(upper limit=1.0, x=w51, lower limit=0.0) -> (coerced(x)=w56:dbl)  [unwired: 1 out]
  n290 = Select(t=w56, s=w52, f=w54) -> (s? t:f=w50:dbl)
  n291 = call <vilib>:"WPI_MotorControlRefNum Registry Get.vi"("refnum name"="Arm Angle Motor") -> ("error out"=w91:errorcluster, "MotorControlDevRef"=w92:T13)  [unwired: 9 in]
  n292 = call <vilib>:"Spark MAX Get Sensor Position.vi"("error in (no error)"=w91, "MotorControlDevRef in"=w92) -> ("error out"=w88:errorcluster, "Sensor Position"=→"Arm Elevation Position":dbl, "MotorControlDevRef out"=w86:T13)  [unwired: 6 in, 1 out]
  n293 = case shown="True" w81 {
    tunnel: [w430 w432] -> w89
    tunnel: w88 -> [w430 w433]
    tunnel: [w429 w431] -> w87
    tunnel: w86 -> [w429 w434]
    frame False {
    }
    frame True {
      n294 = call <vilib>:"Spark MAX Set Sensor Position.vi"("error in"=w433, "MotorControlDeviceRef"=w434) -> ("error out"=w432:errorcluster, "MotorControlDeviceRef"=w431:T13)  [unwired: 8 in]
    }
  }
  n295 = call <vilib>:"CTRE_Phoenix_MotorControl_RefNumRegistryGet.vi"("refnum name"="Arm Tellescope Gearbox Motor") -> ("error out"=w147:errorcluster, "PhoenixMotorControlDevRef"=w148:T13)  [unwired: 9 in]
  n296 = call <vilib>:"CTRE_Phoenix_MotorControl_Set.vi"("error in (no error)"=w147, "Output"=w104, "Control Mode"=w149, "PhoenixMotorControlDevRef"=w148) -> ()  [unwired: 6 in, 2 out]
  n297 = call <vilib>:"WPI_MotorControlSetOutput.vi"("error in (no error)"=w89, "Output"=w50, "MotorControlDevRef"=w87) -> ()  [unwired: 6 in, 3 out]
